vi "Get Relay Position.vi"(8 "error in (no error)":errorcluster, 10 "relay name":string, 11 "SLSC Switch in":refnum<class "SLSC Switch.lvclass">) -> (0 "error out":errorcluster, 2 "position":T1=10 items=["Open"=10, "Closed"=11])   [LabVIEW 2015, in "SLSC Switch.lvclass"]
uses:
  SLSC Switch.lvclass
  Route Manager/Position.ctl
  SLSC Switch.lvclass/SLSC Switch.ctl
  <vilib>/SLSC/Get Device Property (Bool).vi
  <vilib>/SLSC/SLSC.lvlib
  Route Manager/Route Manager.lvclass
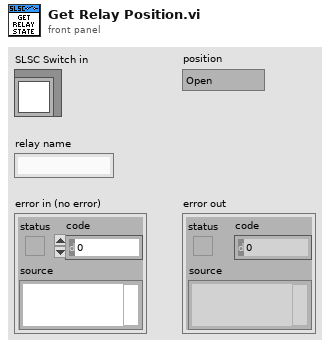
[diagram p1: front panel]
types:
  T1 = typedef "Route Manager.lvclass/Position.ctl" = i32
  T2 = typedef "Route Manager.lvclass/Relay Info.ctl" = cluster{"property":refnum<k21>, "command":refnum<k21>}
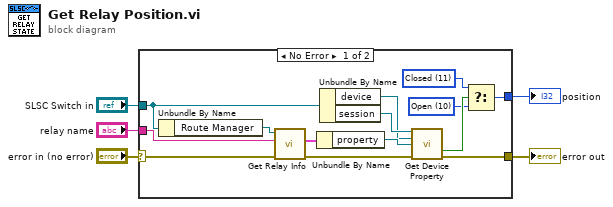
[diagram p0: block diagram]
diagram:
  n1 = case shown="No Error" "error in (no error)" {
    selector: "error in (no error)" -> [w14 w20]
    tunnel: [w12 w20] -> w4
    tunnel: "SLSC Switch in" -> [w19 _]
    tunnel: "relay name" -> [w17 _]
    tunnel: [w8 _] -> w1
    frame No Error {
      w9 = T1 11 items=["Open"=10, "Closed"=11] ("t")
      w10 = T1 10 items=["Open"=10, "Closed"=11] ("position")
      n2 = Unbundle By Name(w19) -> ("Route Manager"=w18:refnum<class "Route Manager.lvclass">)
      n3 = call "Get Relay Info.vi"("error in (no error)"=w14, "relay string"=w17, "Route Manager in"=w18) -> ("error out"=w13:errorcluster, "relay info"=w16:T2)  [unwired: 7 in]
      n4 = Unbundle By Name(w16) -> ("property"=w15:refnum<k21>)
      n5 = Unbundle By Name(w19) -> ("device"=w6:refnum<k21>, "session"=w7:refnum<k21>)
      n6 = call-poly <vilib>:"Get Device Property.vi"("session in"=w7, "devices"=w6, "property"=w15, "error in (no error)"=w13) -> ("property value"=w11:bool, "error out"=w12:errorcluster)  [unwired: 9 in, 1 out]
      n7 = Select(t=w9, s=w11, f=w10) -> (s? t:f=w8:T1)
    }
    frame Error {
    }
  }
  "error out" <- w4
  "position" <- w1
